vi "Initialize.vi"(8 "error in (no error)":errorcluster, 10 "Name":string, 11 "FW Arduino Control in":refnum<class "FW Arduino Control.lvclass">) -> (0 "error out":errorcluster, 3 "FW Arduino Control out":refnum<class "FW Arduino Control.lvclass">)   [LabVIEW 2024, in "FW Arduino Control.lvclass"]
uses:
  FW Arduino Control.lvclass
  C:/Development/Prime-RIMAS/Filter Wheel/Filter Wheel Object/Filter Wheel.lvclass
  FW Arduino Control.lvclass/FW Arduino Control.ctl
  e013e02d-1547-4f39-962f-36d02175e6fd.vi
  Filter Wheel Object/Filter Wheel.lvclass
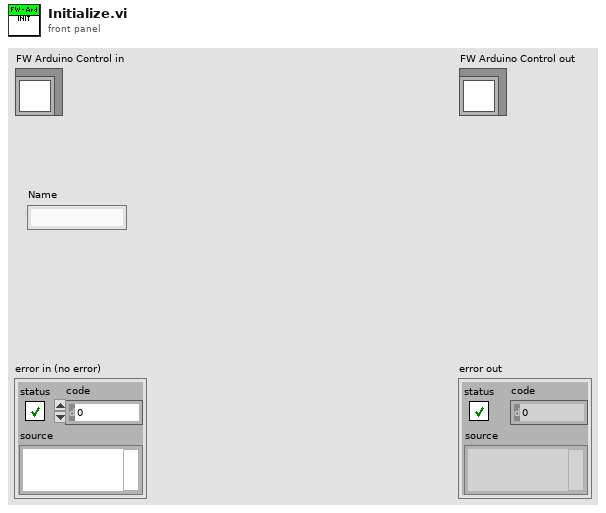
[diagram p1: front panel]
types:
  T1 = typedef "Filter Wheel Arduino Homing cluster.ctl" = cluster{"Direction (F: CW)":bool, "Speed":i32, "Accel":i32, "Min Distance":i32, "Short Leg":i32, "Error Cnts":i32}
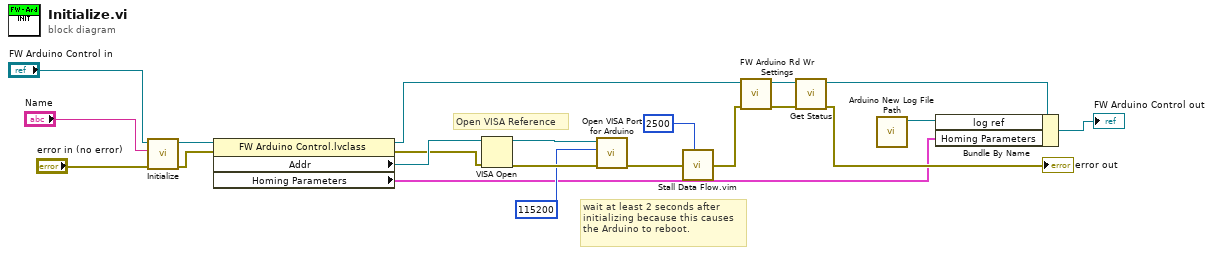
[diagram p0: block diagram]
diagram:
  # "wait at least 2 seconds after initializing because this causes the Arduino to reboot."
  # "Open VISA Reference"
  n1 = call-parent "Initialize.vi"("error in (no error)"="error in (no error)", "Name"="Name", "Filter Wheel in"="FW Arduino Control in") -> ("error out"=w18:errorcluster, "Filter Wheel out"=w19:refnum<class "FW Arduino Control.lvclass">)  [unwired: 7 in]
  n2 = property class="FW Arduino Control.lvclass"(reference=w19, error in=w18) -> (reference out=w9:refnum<class "FW Arduino Control.lvclass">, error out=w16:errorcluster, "Addr"=w17:refnum<visa-resource-name>, "Homing Parameters"=w2:T1)
  n3 = VISA Open(error in (no error)=w16, VISA resource name=w17) -> (VISA resource name=w12:refnum<visa-resource-name>, error out=w13:errorcluster)  [unwired: 3 in]
  n4 = call "Open VISA Port for Arduino.vi"("error in (no error)"=w13, "baud rate (9600)"=u32 115200, "VISA resource name"=w12) -> ("error out"=w10:errorcluster)  [unwired: 7 in, 1 out]
  n5 = call "Stall Data Flow.vim"("value in"=w10, "milliseconds to wait"=u32 2500) -> ("value out"=w8:errorcluster)  [unwired: 1 out]
  n6 = call "FW Arduino Rd Wr Settings.vi"("error in (no error)"=w8, "Settings"=w9) -> ("error out"=w4:errorcluster, "Settings"=w6:refnum<class "FW Arduino Control.lvclass">)  [unwired: 8 in]
  n7 = call-dynamic "Get Status.vi"("error in (no error)"=w4, "FW Arduino Control in"=w6) -> ("error out"=→"error out":errorcluster, "FW Arduino Control out"=w5:refnum<class "FW Arduino Control.lvclass">)  [unwired: 7 in, 1 out]
  n8 = call "Arduino New Log File Path.vi"() -> ("log ref"=w7:refnum<file>)  [unwired: 11 in]
  n9 = Bundle By Name(cluster=w5, "log ref"=w7, "Homing Parameters"=w2) -> (→"FW Arduino Control out":refnum<class "FW Arduino Control.lvclass">)
